vi "Wärmestromrechner.vi"(3 "Taus":dbl, 4 "Tein":dbl, 5 "Massenstrom":dbl) -> (1 "Wärmestrom Q":dbl)   [LabVIEW 2015]
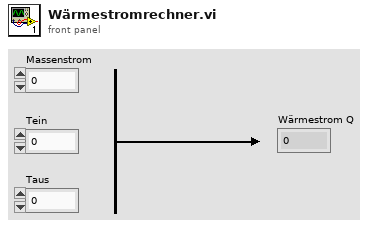
[diagram p1: front panel]
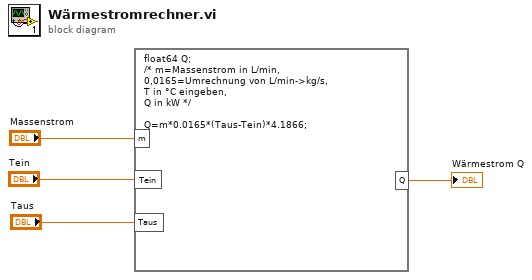
[diagram p0: block diagram]
diagram:
  n1 = formula code="float64 Q;\n/* m=Massenstrom in L/min, \n0,0165=Umrechnung von L/min->kg/s,\nT in °C eingeben, \nQ in kW */\n\nQ=m*0.0165*(Taus-Tein)*4.1866;"("m"="Massenstrom", "Taus"="Taus", "Tein"="Tein") -> ("Q"=→"Wärmestrom Q":dbl)
